vi "2041_RS232_interface.vi"() -> ()   [LabVIEW 2010]
uses:
  <vilib>/Instr/_visa.llb/VISA Configure Serial Port (Instr).vi
panel:
  in  "Boolean":bool
  in  "stop":bool
  out "number":i32
  out "substring 2":string
  out "substring":string
  out "status":string
  out "time":string
  out "resistance":string
  out "current":string
  out "voltage":string
  in  "delay (ms)":u32=500
  out "Bytes at Port":u32
  out "read buffer":string
  in  "write buffer":string="meas?\n"
  in  "flow control (0:none)":u16(ring) items=["None", "XON/XOFF", "RTS/CTS", "XON/XOFF & RTS/CTS", "DTR/DSR", "XON/XOFF & DTR/DSR"]
  in  "stop bits (10: 1 bit)":u16(ring)=10 items=["1.0"=10, "1.5"=15, "2.0"=20]
  in  "parity (0:none)":enum16{"None", "Odd", "Even", "Mark", "Space"}(ring)
  in  "data bits (8)":u16=8 min=5 max=8 step=1
  in  "baud rate (9600)":u32=9600
  in  "VISA Port":refnum<visa-resource-name>="COM1"
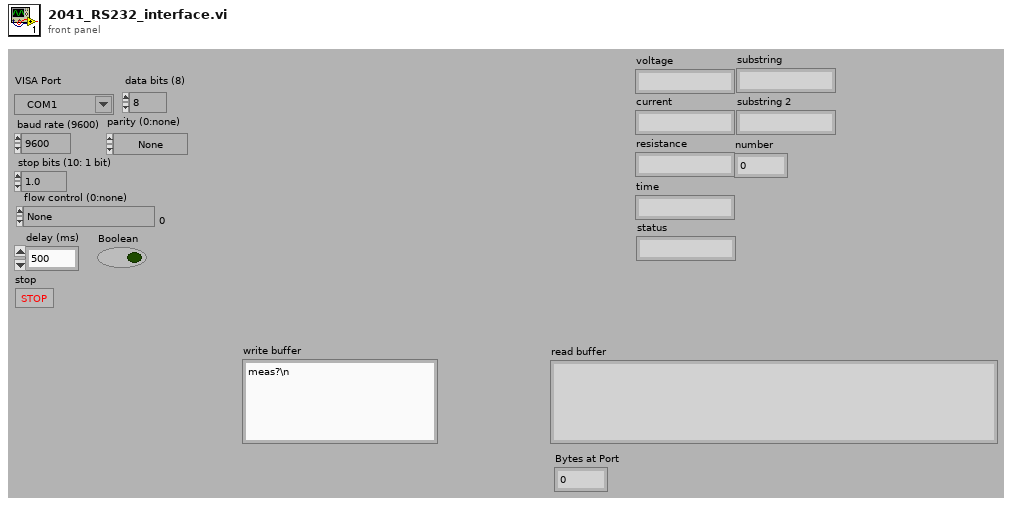
[diagram p1: front panel]
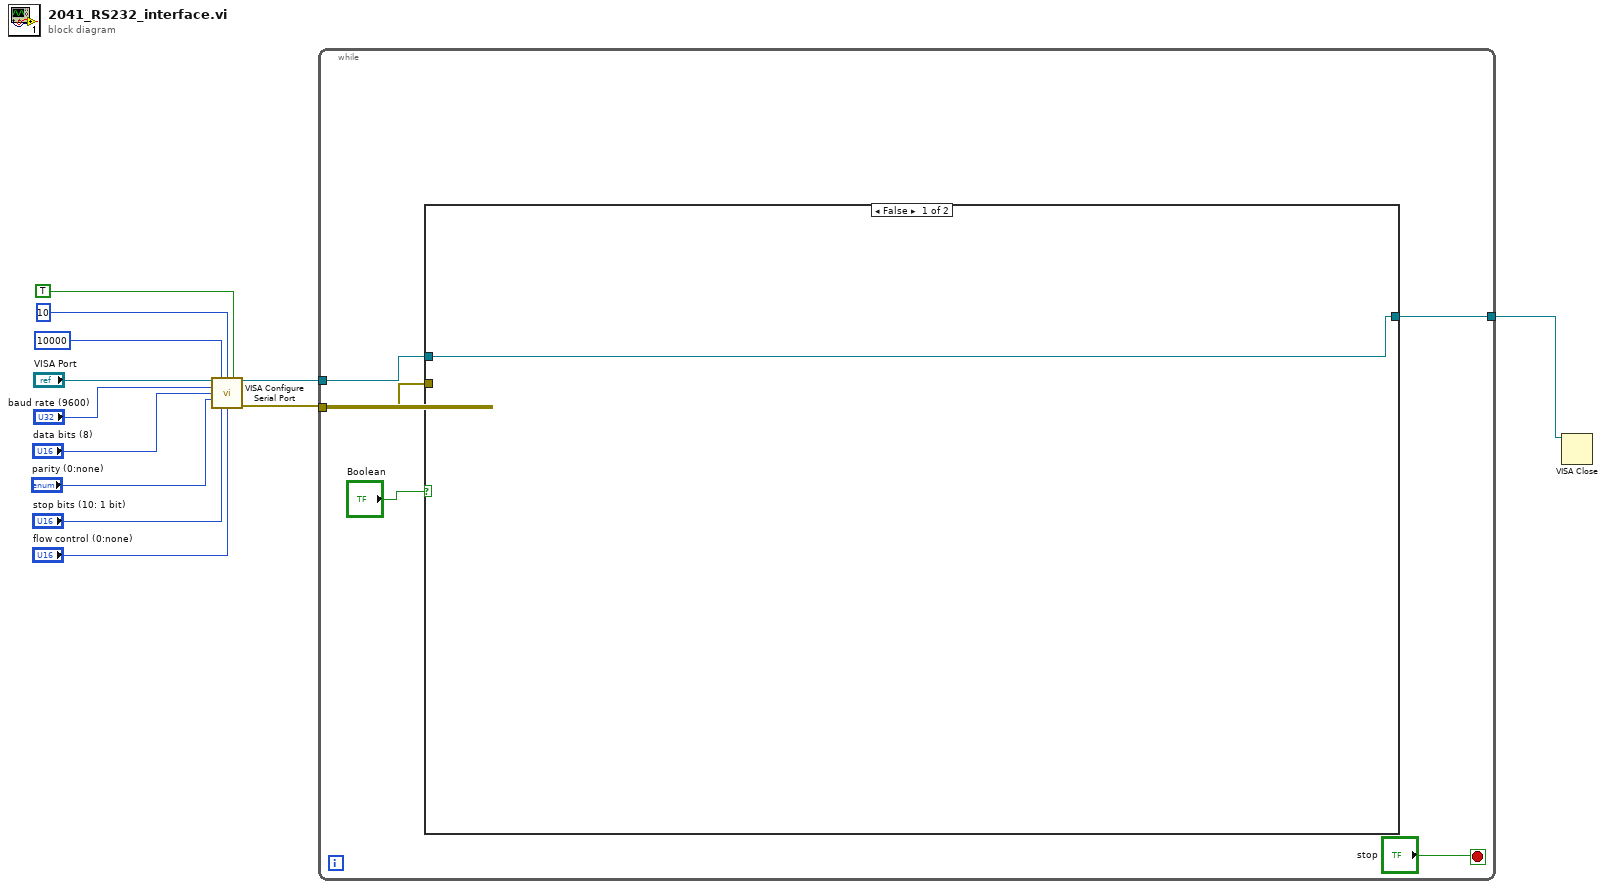
[diagram p0: block diagram]
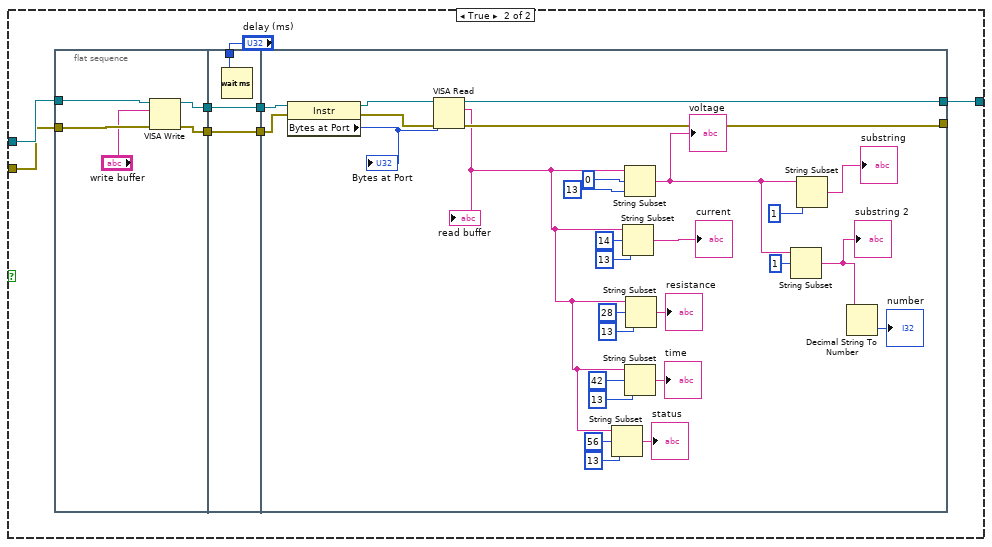
[diagram p2: hidden frame]
diagram:
  n1 = call-poly "VISA Configure Serial Port"("VISA resource name"="VISA Port", "timeout (10sec)"=u32 10000, "termination char\n(0xA = '\\n' = LF)"=u8 10 ("termination char\n(0xA = '\\n' = LF)"), "Enable Termination\nChar (T)"=TRUE ("Enable Termination\nChar (T)"), "baud rate (9600)"="baud rate (9600)", "data bits (8)"="data bits (8)", "parity (0:none)"="parity (0:none)", "stop bits (10: 1 bit)"="stop bits (10: 1 bit)", "flow control (0:none)"="flow control (0:none)") -> ("VISA resource name out"=w3:refnum<visa-resource-name>, "error out"=w2:errorcluster)  [unwired: 5 in]
  n2 = while {
    tunnel: w3 -> [w17]
    tunnel: w2 -> [w16]
    tunnel: [w13] -> w1
    stop <- "stop" stop-if-true
    n3 = case shown="False" "Boolean" {
      tunnel: w17 -> [w18 w22]
      tunnel: w16 -> [_ w21]
      tunnel: [w18 w19] -> w13
      frame False {
      }
      frame True {
        n4 = flat-sequence {
          tunnel: w22 -> [w31]
          tunnel: w21 -> [w30]
          tunnel: [w28] -> w26
          tunnel: [w27] -> w25
          tunnel: w26 -> [w34]
          tunnel: [w34] -> w24
          tunnel: w25 -> [w33]
          tunnel: [w33] -> w23
          tunnel: "delay (ms)" -> [w32]
          tunnel: w24 -> [w59]
          tunnel: [w58] -> _
          tunnel: w23 -> [w57]
          tunnel: [w35] -> w19
          frame #0 {
            n5 = VISA Write(VISA resource name=w31, write buffer="write buffer", error in (no error)=w30) -> (VISA resource name out=w28:refnum<visa-resource-name>, error out=w27:errorcluster)  [unwired: 1 out]
          }
          frame #1 {
            n6 = Wait (ms)(milliseconds to wait=w32) -> ()  [unwired: 1 out]
          }
          frame #2 {
            n7 = property class="Instr"(reference=w59, error in=w57) -> (reference out=w61:refnum<visa-resource-name>, error out=w60:errorcluster, "Bytes at Port"=w62:u32)
            "Bytes at Port" <- w62
            n8 = VISA Read(VISA resource name=w61, byte count=w62, error in (no error)=w60) -> (VISA resource name out=w35:refnum<visa-resource-name>, read buffer=w45:string, error out=w58:errorcluster)  [unwired: 1 out]
            "read buffer" <- w45
            n9 = String Subset(string=w45, offset (0)=56, length (rest)=13 ("length (rest)")) -> (substring=→"status":string)
            n10 = String Subset(string=w45, offset (0)=14, length (rest)=13 ("length (rest)")) -> (substring=→"current":string)
            n11 = String Subset(string=w45, offset (0)=0, length (rest)=13 ("length (rest)")) -> (substring=w39:string)
            "voltage" <- w39
            n12 = String Subset(string=w45, offset (0)=42, length (rest)=13 ("length (rest)")) -> (substring=→"time":string)
            n13 = String Subset(string=w45, offset (0)=28, length (rest)=13 ("length (rest)")) -> (substring=→"resistance":string)
            n14 = String Subset(string=w39, offset (0)=1) -> (substring=w37:string)  [unwired: 1 in]
            "substring 2" <- w37
            n15 = String Subset(string=w39, length (rest)=1 ("length (rest)")) -> (substring=→"substring":string)  [unwired: 1 in]
            n16 = Decimal String To Number(string=w37) -> (number=→"number":i32)  [unwired: 2 in, 1 out]
          }
        }
      }
    }
  }
  n17 = VISA Close(VISA resource name=w1) -> ()  [unwired: 1 in, 1 out]
